vi "Write Conversion Time.vi"(8 "error in":errorcluster, 10 "Conversion Time":T1 items=["High Speed (1k S/s)", "Medium Speed (100 S/s)", "Medium Resolution (50/60Hz Rejection - 12 S/s)", "High Resolution (50/60Hz rejection - 2 S/s)"], 11 "9224 in":refnum<class "9224.lvclass">) -> (0 "error out":errorcluster, 3 "9224 out":refnum<class "9224.lvclass">)   [LabVIEW 2017, in "Modules.lvlib" / "9224.lvclass"]
uses:
  9224.lvclass
  Conversion Time.ctl
  9224.lvclass/9224.ctl
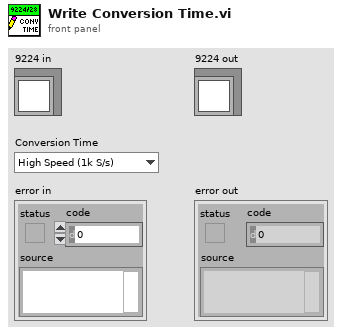
[diagram p1: front panel]
types:
  T1 = typedef "Modules.lvlib/9224.lvclass/Conversion Time.ctl" = u16
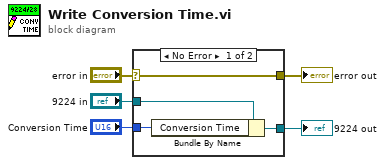
[diagram p0: block diagram]
diagram:
  n1 = case shown="No Error" "error in" {
    selector: "error in" -> [w9 w10]
    tunnel: [w9 w10] -> w4
    tunnel: [w7 w11] -> w2
    tunnel: "9224 in" -> [w8 w11]
    tunnel: "Conversion Time" -> [w6 _]
    frame No Error {
      n2 = Bundle By Name(cluster=w8, "Conversion Time"=w6) -> (w7:refnum<class "9224.lvclass">)
    }
    frame Error {
    }
  }
  "error out" <- w4
  "9224 out" <- w2
